vi "Flight Gear Data Initialization VI.vi"(8 "error in (no error)":errorcluster, 10 "Custom XML":string, 11 "Device Item Ref in":T1 format="%.0x") -> (0 "error out":errorcluster, 3 "Device Item Ref out":T1 format="%.0x")   [LabVIEW 2010, in "Flight Gear Data Custom Device.lvlib"]
uses:
  Flight Gear Data Custom Device.lvlib
  <vilib>/NI VeriStand/Custom Device API/Custom Device Item Ref.ctl
  <vilib>/NI VeriStand/Custom Device API/Custom Device Channel.ctl
  <vilib>/NI VeriStand/Custom Device API/Custom Device Channel Type.ctl
  <vilib>/NI Veristand/Custom Device API/Custom Device Loop Type.ctl
  <vilib>/NI Veristand/Custom Device API/Custom Device API.lvlib
panel:
  in  "Channels":string[](array[string])=["Version", "Longitude", "Latitude", "Altitude", "Above Ground Level", "Phi", "Theta", "Psi", "Alpha", "Beta", "Phidot", "Thetadot", "Psidot", "Vcas", "Climb Rate", "V North", "V East", "V Down", "V Wind Body North", "V Wind Body East", "V Wind Body Down", "Acceleration X Pilot", "Acceleration Y Pilot", "Acceleration Z Pilot", "Stall Warning", "Slip Ball Deflection", "Number of Engines", "Engine 0 State", "Engine 1 State", "Engine 2 State", "Engine 3 State", "Engine 0 RPM", "Engine 1 RPM", "Engine 2 RPM", "Engine 3 RPM", "Engine 0 Fuel Flow", "Engine 1 Fuel Flow", "Engine 2 Fuel Flow", "Engine 3 Fuel Flow", "Engine 0 Fuel Pressure", "Engine 1 Fuel Pressure", "Engine 2 Fuel Pressure", "Engine 3 Fuel Pressure", "Engine 0 Exhaust Gas Temp", "Engine 1 Exhaust Gas Temp", "Engine 2 Exhaust Gas Temp", "Engine 3 Exhaust Gas Temp", "Engine 0 Cylinder Head Temp", "Engine 1 Cylinder Head Temp", "Engine 2 Cylinder Head Temp", "Engine 3 Cylinder Head Temp", "Engine 0 Manifold Pressure", "Engine 1 Manifold Pressure", "Engine 2 Manifold Pressure", "Engine 3 Manifold Pressure", "Engine 0 Turbine Inlet Temperature", "Engine 1 Turbine Inlet Temperature", "Engine 2 Turbine Inlet Temperature", "Engine 3 Turbine Inlet Temperature", "Engine 0 Oil Temp", "Engine 1 Oil Temp", "Engine 2 Oil Temp", "Engine 3 Oil Temp", "Engine 0 Oil Pressure", "Engine 1 Oil Pressure", "Engine 2 Oil Pressure", "Engine 3 Oil Pressure", "Number of Tanks", "Tank 0 Fuel Quantity", "Tank 1 Fuel Quantity", "Tank 2 Fuel Quantity", "Tank 3 Fuel Quantity", "Current Time", "Time Offset", "Visibility", "Elevator", "Elevator Trim Tab", "Left Flap", "Right Flap", "Left Aileron", "Right Aileron", "Rudder", "Nose Wheel", "Speedbrake", "Spoilers"]
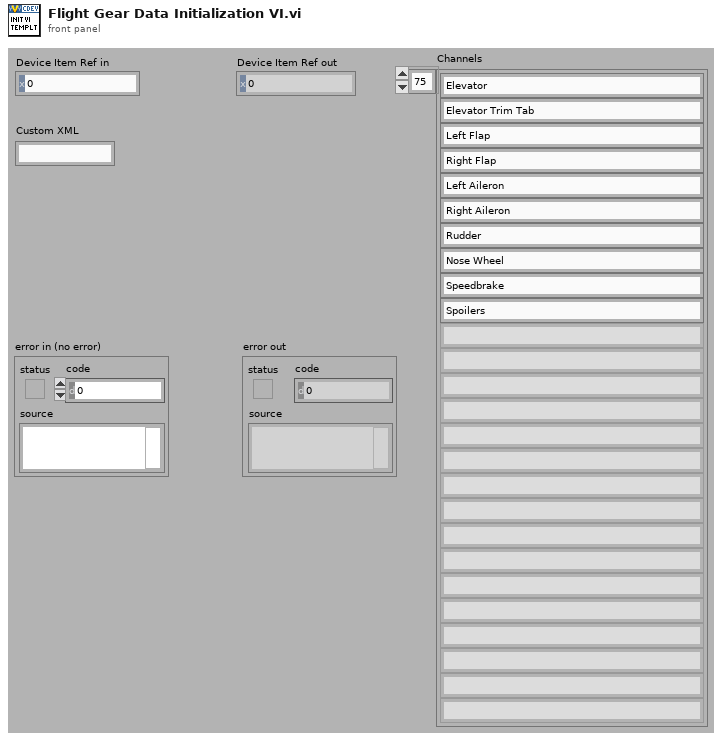
[diagram p1: front panel]
types:
  T1 = typedef "Custom Device API.lvlib/Custom Device Item Ref.ctl" = u64
  T2 = typedef "Custom Device API.lvlib/Custom Device Channel.ctl" = cluster{"Type":T3, "Units":string, "Default Value":dbl, "Faultable":bool, "Scalable":bool}
  T3 = typedef "Custom Device API.lvlib/Custom Device Channel Type.ctl" = enum16{"Input", "Output"}
  T4 = typedef "Custom Device API.lvlib/Custom Device Loop Type.ctl" = enum32{"While Loop", "Timed Loop"}
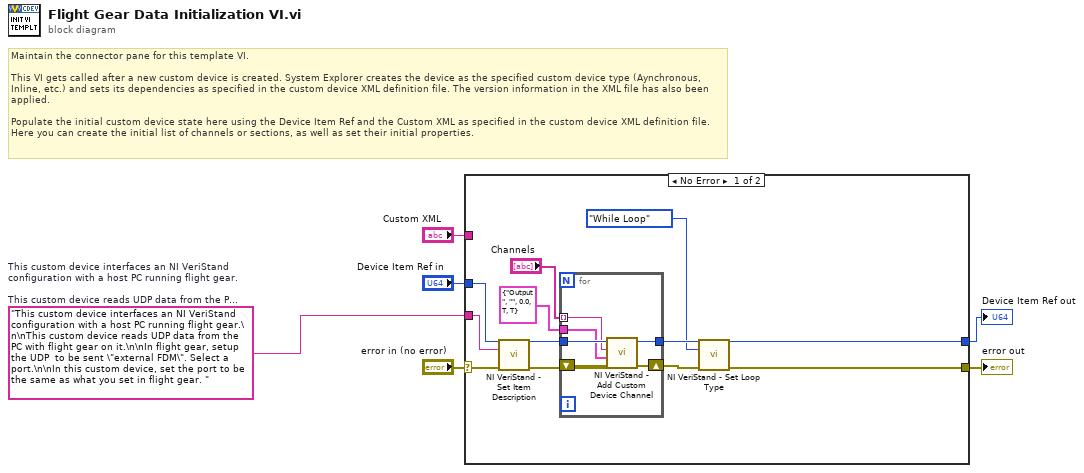
[diagram p0: block diagram]
diagram:
  w1 = "This custom device interfaces an NI VeriStand configuration with a host PC running flight gear.\n\nThis custom device reads UDP data from the PC with flight gear on it.\n\nIn flight gear, setup the UDP  to be sent \"external FDM\". Select a port.\n\nIn this custom device, set the port to be the same as what you set in flight gear. "  # This custom device interfaces an NI VeriStand configuration with a host PC running flight gear.  This custom device reads UDP data from the PC with flight gear on it.  In flight gear, setup the UDP  to be sent "external FDM". Select a port.  In this custom device, set the port to be the same as what you set in flight gear.
  # "Maintain the connector pane for this template VI.\n\nThis VI gets called after a new custom device is created. System Explorer creates the device as the specified custom device type (Aynchronous, Inline, etc.) and sets its dependencies as specified in the custom device XML definition file. The version information in the XML file has also been applied.\n\nPopulate the initial custom device state here using the Device Item Ref and the Custom XML as specified in the custom device XML definition file. Here you can create the initial list of channels or sections, as well as set their initial properties."
  n1 = case shown="No Error" "error in (no error)" {
    selector: "error in (no error)" -> [w17 w26]
    tunnel: [w8 w26] -> w6
    tunnel: [w7 w25] -> w4
    tunnel: "Device Item Ref in" -> [w18 w25]
    tunnel: "Custom XML" -> [_ _]
    tunnel: w1 -> [w16 _]
    frame No Error {
      n2 = call <vilib>:"NI VeriStand - Set Item Description.vi"("error in (no error)"=w17, "Description"=w16, "Item Ref in"=w18) -> ("error out"=w15:errorcluster, "Item Ref out"=w14:T1)  [unwired: 6 in, 1 out]
      n3 = for {
        tunnel: w14 -> [w23]
        tunnel: "Channels" -> [w22] mode=indexing
        tunnel: T2 {"Type"=enum."Output", "Units"="", "Default Value"=0.0, "Faultable"=TRUE, "Scalable"=TRUE} ("Channel") -> [w21]
        shift-right: [w20] -> w11
        shift-left: w15 -> [w24]
        tunnel: [w19] -> w10
        n4 = call <vilib>:"NI VeriStand - Add Custom Device Channel.vi"("error in (no error)"=w24, "Channel"=w21, "Channel Name"=w22, "Parent Ref in"=w23) -> ("error out"=w20:errorcluster, "Parent Ref out"=w19:T1)  [unwired: 4 in, 2 out]
      }
      n5 = call <vilib>:"NI VeriStand - Set Loop Type.vi"("error in (no error)"=w11, "Loop type"=Custom_Device_Loop_Type."While Loop", "Device Ref in"=w10) -> ("error out"=w8:errorcluster, "Device Ref out"=w7:T1)  [unwired: 7 in]
    }
    frame Error {
    }
  }
  "error out" <- w6
  "Device Item Ref out" <- w4
